vi "Premade windows.vi"() -> (2 "Premade Windows (pic)":picture[](array[picture]), 3 "Premade Windows":cluster{"Plot Bounds":T1[]}[](array[cluster]) {"Plot Bounds"."Plot Bounds (%)"."Bottom (%)" format="%.2f"; "Plot Bounds"."Plot Bounds (%)"."Top (%)" format="%.2f"; "Plot Bounds"."Plot Bounds (%)"."Right (%)" format="%.2f"; "Plot Bounds"."Plot Bounds (%)"."Left (%)" format="%.2f"})   [LabVIEW 2021, in "MultiStokePlot.lvlib" / "MultiPlotPanel.lvclass"]
uses:
  Classes/MultiPlotPanel/MultiPlotPanel.lvclass
  Window Position and plot number.ctl
  Window Position.ctl
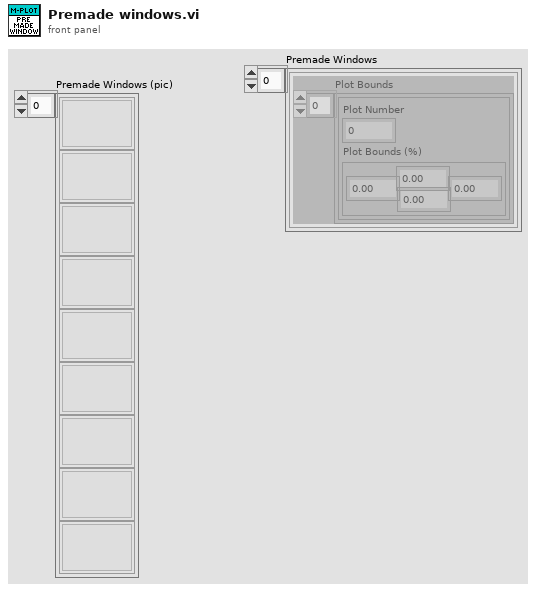
[diagram p1: front panel]
types:
  T1 = typedef "MultiStokePlot.lvlib/MultiPlotPanel.lvclass/Window Position and plot number.ctl" = cluster{"Plot Number":i32, "Plot Bounds (%)":T2}
  T2 = typedef "MultiStokePlot.lvlib/MultiPlotPanel.lvclass/Window Position.ctl" = cluster{"Left (%)":dbl, "Top (%)":dbl, "Right (%)":dbl, "Bottom (%)":dbl}
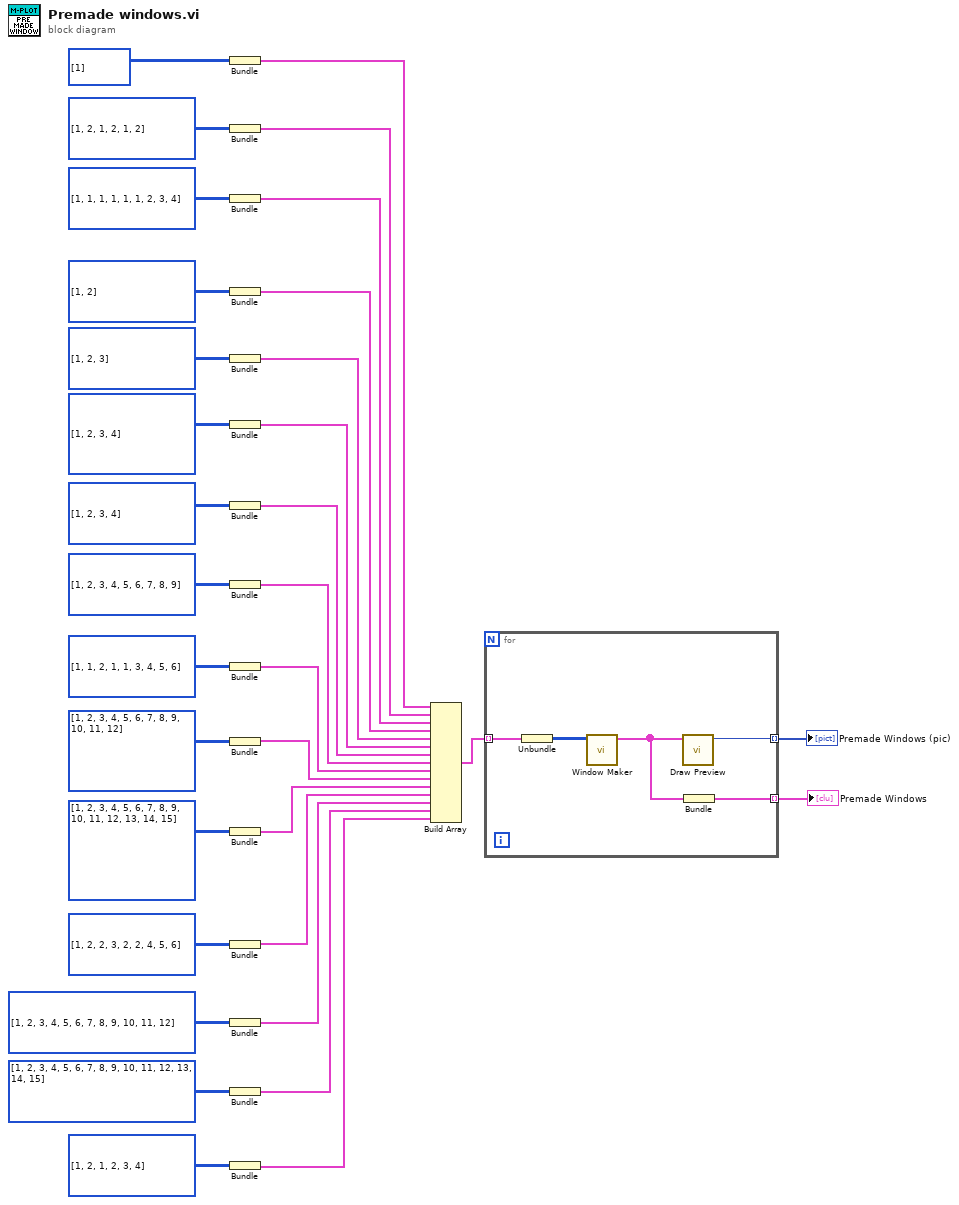
[diagram p0: block diagram]
diagram:
  n1 = Bundle("1 plot"=i32[][] [[1]]) -> (w24:cluster{"1 plot":i32[][]})  [unwired: 1 in]
  n2 = Bundle("9 plot"=i32[][] [[1, 2], [1, 2], [1, 2]]) -> (w15:cluster{"9 plot":i32[][]})  [unwired: 1 in]
  n3 = Bundle("9 plot"=i32[][] [[1, 1, 1], [1, 1, 1], [2, 3, 4]]) -> (w14:cluster{"9 plot":i32[][]})  [unwired: 1 in]
  n4 = Bundle("9 plot"=i32[][] [[1], [2]]) -> (w13:cluster{"9 plot":i32[][]})  [unwired: 1 in]
  n5 = Bundle("9 plot"=i32[][] [[1], [2], [3]]) -> (w12:cluster{"9 plot":i32[][]})  [unwired: 1 in]
  n6 = Bundle("9 plot"=i32[][] [[1], [2], [3], [4]]) -> (w11:cluster{"9 plot":i32[][]})  [unwired: 1 in]
  n7 = Bundle("4 plot"=i32[][] [[1, 2], [3, 4]]) -> (w10:cluster{"4 plot":i32[][]})  [unwired: 1 in]
  n8 = Bundle("9 plot"=i32[][] [[1, 2, 3], [4, 5, 6], [7, 8, 9]]) -> (w9:cluster{"9 plot":i32[][]})  [unwired: 1 in]
  n9 = Bundle("9 plot"=i32[][] [[1, 1, 2], [1, 1, 3], [4, 5, 6]]) -> (w8:cluster{"9 plot":i32[][]})  [unwired: 1 in]
  n10 = Bundle("9 plot"=i32[][] [[1, 2, 3], [4, 5, 6], [7, 8, 9], [10, 11, 12]]) -> (w18:cluster{"9 plot":i32[][]})  [unwired: 1 in]
  n11 = Bundle("9 plot"=i32[][] [[1, 2, 3], [4, 5, 6], [7, 8, 9], [10, 11, 12], [13, 14, 15]]) -> (w17:cluster{"9 plot":i32[][]})  [unwired: 1 in]
  n12 = Bundle("9 plot"=i32[][] [[1, 2, 2], [3, 2, 2], [4, 5, 6]]) -> (w1:cluster{"9 plot":i32[][]})  [unwired: 1 in]
  n13 = Bundle("9 plot"=i32[][] [[1, 2, 3, 4], [5, 6, 7, 8], [9, 10, 11, 12]]) -> (w5:cluster{"9 plot":i32[][]})  [unwired: 1 in]
  n14 = Bundle("9 plot"=i32[][] [[1, 2, 3, 4, 5], [6, 7, 8, 9, 10], [11, 12, 13, 14, 15]]) -> (w4:cluster{"9 plot":i32[][]})  [unwired: 1 in]
  n15 = Bundle("9 plot"=i32[][] [[1, 2], [1, 2], [3, 4]]) -> (w3:cluster{"9 plot":i32[][]})  [unwired: 1 in]
  n16 = Build Array(w24, w15, w14, w13, w12, w11, w10, w9, w8, w18, w17, w1, w5, w4, w3) -> (w30:cluster{"9 plot":i32[][]}[])
  n17 = for {
    tunnel: w30 -> [w38] mode=indexing
    tunnel: [w36] -> w29 mode=indexing
    tunnel: [w34] -> w21 mode=indexing
    n18 = Unbundle(w38) -> ("9 plot"=w37:i32[][])
    n19 = call "Window Maker.vi"("Simple Windows"=w37) -> ("Plot Bounds"=w35:T1[])  [unwired: 10 in]
    n20 = call "Draw Preview.vi"("Plot Bounds"=w35) -> ("Preview Pict"=w36:picture)  [unwired: 10 in]
    n21 = Bundle("Plot Bounds"=w35) -> (w34:cluster{"Plot Bounds":T1[]})  [unwired: 1 in]
  }
  "Premade Windows (pic)" <- w29
  "Premade Windows" <- w21
